vi "logThermal.vi"(6 "Temp Readings":T1 {"Ambient Temp (°F)" format="%.2f °F"; "Ambient Temp (°C)" format="%.2f °C"; "Object Temp (°F)" format="%.2f °F"; "Object Temp (°C)" format="%.2f °C"}, 8 "Online":bool, 9 "Index":i32) -> ()   [LabVIEW 2017]
uses:
  Type Defs/tempReadings.ctl
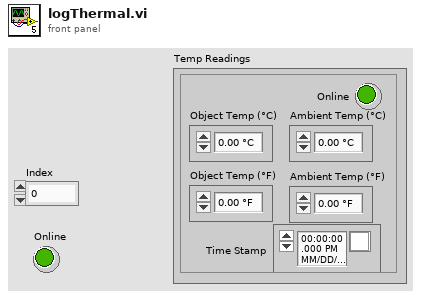
[diagram p1: front panel]
types:
  T1 = typedef "tempReadings.ctl" = cluster{"Object Temp (°C)":dbl, "Object Temp (°F)":dbl, "Ambient Temp (°C)":dbl, "Ambient Temp (°F)":dbl, "Online":bool, "Time Stamp":timestamp}
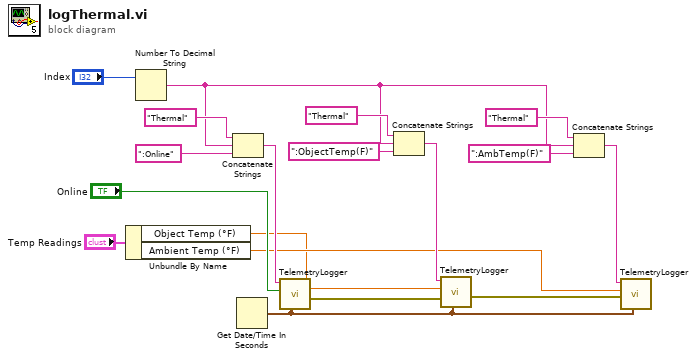
[diagram p0: block diagram]
diagram:
  n1 = Unbundle By Name("Temp Readings") -> ("Object Temp (°F)"=w3:dbl, "Ambient Temp (°F)"=w4:dbl)
  n2 = Number To Decimal String(number="Index") -> (decimal integer string=w7:string)  [unwired: 1 in]
  n3 = Concatenate Strings("Thermal", w7, ":Online") -> (w14:string)
  n4 = Get Date/Time In Seconds() -> (seconds since 1Jan1904=w6:timestamp)
  n5 = call "TelemetryLogger.vi"("Time Stamp"=w6, "Data"="Online", "Sensor:Reading"=w14) -> ("Error Out"=w2:errorcluster)  [unwired: 8 in]
  n6 = Concatenate Strings("Thermal", w7, ":ObjectTemp(F)") -> (w13:string)
  n7 = call "TelemetryLogger.vi"("Time Stamp"=w6, "Error In"=w2, "Data"=w3, "Sensor:Reading"=w13) -> ("Error Out"=w1:errorcluster)  [unwired: 7 in]
  n8 = Concatenate Strings("Thermal", w7, ":AmbTemp(F)") -> (w8:string)
  n9 = call "TelemetryLogger.vi"("Time Stamp"=w6, "Error In"=w1, "Data"=w4, "Sensor:Reading"=w8) -> ()  [unwired: 7 in, 1 out]
